vi "Sequence Timout--constant.vi"() -> (0 "Sequence Timeout (ms)":i32=5000)   [LabVIEW 2024, in "Auto Modo.lvlib"]
uses:
  Auto Modo.lvlib
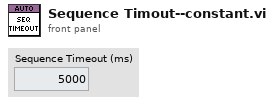
[diagram p1: front panel]
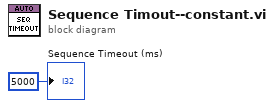
[diagram p0: block diagram]
diagram:
  "Sequence Timeout (ms)" <- 5000
